vi "Tenerowicz_B_1.vi"   [LabVIEW 2020]
uses:
  <vilib>/Platform/TimedLoop/XDataNode/timing_clust.ctl
  <vilib>/Platform/TimedLoop/XDataNode/nitl_modes.ctl
  <vilib>/Platform/TimedLoop/XDataNode/wakeup.ctl
  <vilib>/platform/TimedLoop/XDataNode/XDataNode.xnode
  <vilib>/Platform/TimedLoop/XDataNode/XDNodeRunTimeDep.lvlib
types:
  T1 = typedef "Rendezvous RefNum" = refnum<k1>
  T2 = typedef "Semaphore RefNum" = refnum<k1>
  T3 = typedef "XDNodeRunTimeDep.lvlib/timing_clust.ctl" = cluster{"Expected End [f-1]":u64, "Actual End [f-1]":u64, "Finished Late? [f-1]":bool, "Expected End [i-1]":u64, "Actual End [i-1]":u64, "Finished Late? [i-1]":bool, "Expected Start [i]":u64, "Actual Start [i]":u64, "Expected Start [f]":u64, "Actual Start [f]":u64, "Source Name":string, "Structure Name":string, "Period":i64, "Deadline":i64, "Offset":i64, "Start":i64, "Priority":i32, "Timeout":i32, "Mode":T4, "Wakeup Reason":T5, "Error":errorcluster, "Source Type":string, "Secondary Source Type":string, "Global End Time":u64, "Global Start Time":u64, "Frame Duration":u64, "Iteration Duration":u64, "Assigned CPU":i32, "I/O Scan Engine Mode":u32}
  T4 = typedef "XDNodeRunTimeDep.lvlib/nitl_modes.ctl" = enum32{"No Change", "Process missed periods, maintain original phase", "Discard missed periods, maintain original phase", "Process missed periods, ignore original phase", "Discard missed periods, ignore original phase"}
  T5 = typedef "XDNodeRunTimeDep.lvlib/wakeup.ctl" = enum32{"Normal", "Aborted", "Asynchronous wakeup", "Timing source error", "Timed loop error", "Timeout"}
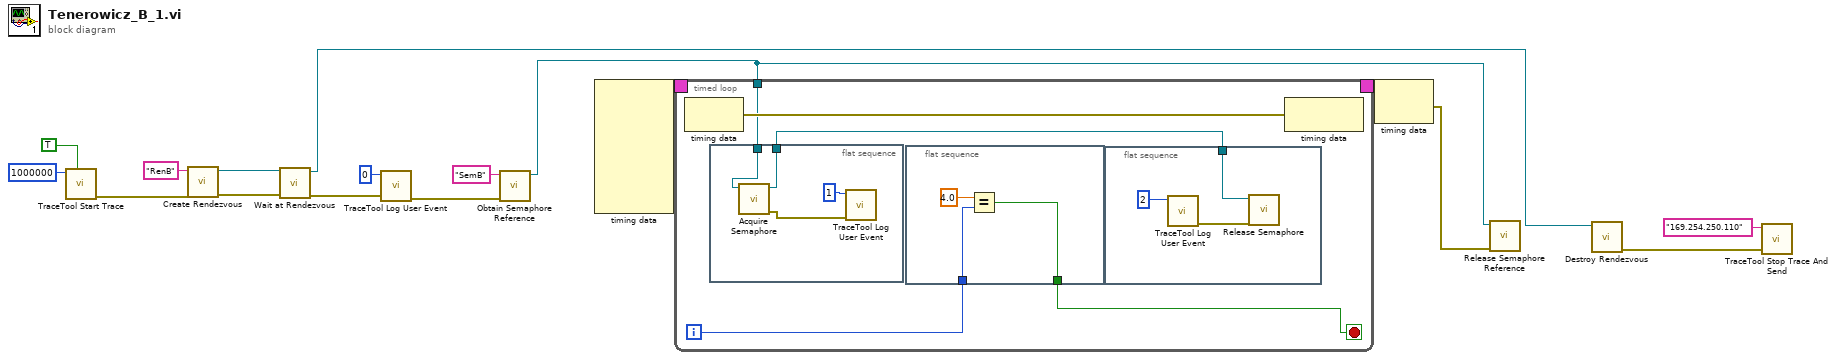
[diagram p0: block diagram]
diagram:
  n1 = call <vilib>:"TraceTool Start Trace.vi"("Detailed Tracing? (F)"=TRUE, "Buffer Size (250000 bytes)"=1000000) -> ("error out"=w8:errorcluster)  [unwired: 8 in, 1 out]
  n2 = call <vilib>:"Create Rendezvous.vi"("error in (no error)"=w8, "name (unnamed)"="RenB") -> ("error out"=w7:errorcluster, "rendezvous"=w9:T1)  [unwired: 3 in, 1 out]
  n3 = call <vilib>:"Wait at Rendezvous.vi"("error in (no error)"=w7, "rendezvous"=w9) -> ("error out"=w6:errorcluster, "rendezvous out"=w3:T1)  [unwired: 3 in, 1 out]
  n4 = call <vilib>:"TraceTool Log User Event.vi"("error in (no error)"=w6, "Event ID (0-255)"=u32 0) -> ("error out"=w5:errorcluster)  [unwired: 9 in]
  n5 = call <vilib>:"Obtain Semaphore Reference.vi"("error in (no error)"=w5, "name (unnamed)"="SemB") -> ("semaphore"=w4:T2)  [unwired: 3 in, 2 out]
  n6 = node-c288() -> (w17:T3)  [unwired: 7 in]
  n7 = timed-loop {
    timing: w17 -> [_]
    timing-out: [_] -> w16
    tunnel: w4 -> [w19]
    i -> [w21]
    stop <- w20 stop-if-true
    n8 = node-c288() -> (w22:errorcluster)  [unwired: 1 in]
    n9 = flat-sequence {
      tunnel: w19 -> [w31]
      tunnel: [w30] -> w18
      frame #0 {
        n10 = call <vilib>:"Acquire Semaphore.vi"("semaphore"=w31) -> ("error out"=w29:errorcluster, "semaphore out"=w30:T2)  [unwired: 4 in, 1 out]
        n11 = call <vilib>:"TraceTool Log User Event.vi"("error in (no error)"=w29, "Event ID (0-255)"=u32 1) -> ()  [unwired: 9 in, 1 out]
      }
    }
    n12 = flat-sequence {
      tunnel: w21 -> [w27]
      tunnel: [w26] -> w20
      frame #0 {
        n13 = Equal?(x=4.0, y=w27) -> (x = y?=w26:bool)
      }
    }
    n14 = flat-sequence {
      tunnel: w18 -> [w24]
      frame #0 {
        n15 = call <vilib>:"TraceTool Log User Event.vi"("Event ID (0-255)"=u32 2) -> ("error out"=w23:errorcluster)  [unwired: 10 in]
        n16 = call <vilib>:"Release Semaphore.vi"("error in (no error)"=w23, "semaphore"=w24) -> ()  [unwired: 4 in, 2 out]
      }
    }
    n17 = node-c288(w22) -> ()  [unwired: 1 out]
  }
  n18 = node-c288(w16) -> (w2:errorcluster)
  n19 = call <vilib>:"Release Semaphore Reference.vi"("error in (no error)"=w2, "semaphore"=w4) -> ()  [unwired: 8 in, 2 out]
  n20 = call <vilib>:"Destroy Rendezvous.vi"("rendezvous"=w3) -> ("error out"=w1:errorcluster)  [unwired: 5 in, 1 out]
  n21 = call <vilib>:"TraceTool Stop Trace And Send.vi"("error in (no error)"=w1, "Trace Host Network Address"="169.254.250.110") -> ()  [unwired: 9 in, 1 out]
